vi "LaserToBuffer.vi"() -> ()   [LabVIEW 2016]
uses:
  <instrlib>/Keyence LK-G3000/Public/clusters/LKIF_FLOATVALUE.ctl
  <instrlib>/Keyence LK-G3000/Public/enums/LKIF_FLOATRESULT.ctl
  <instrlib>/Keyence LK-G3000/Keyence LK-G3000.lvlib
panel:
  in  "timing":u32=500
  out "Measurements":dbl[][](array[numeric])
  out "CalcData2":T1 {"LKIF_FLOATRESULT" items=["VALID", "RANGEOVER_P", "RANGEOVER_N", "WAITING"]}
  out "CalcData1":T1 {"LKIF_FLOATRESULT" items=["VALID", "RANGEOVER_P", "RANGEOVER_N", "WAITING"]}
  in  "Stop VI":bool
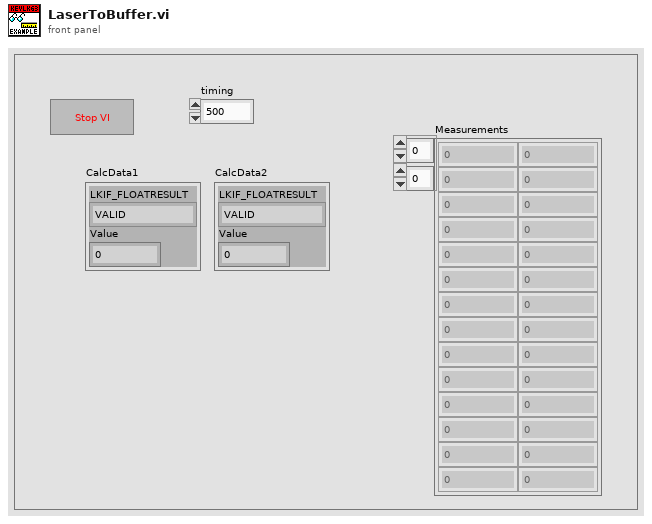
[diagram p1: front panel]
types:
  T1 = typedef "Keyence LK-G3000.lvlib/LKIF_FLOATVALUE.ctl" = cluster{"LKIF_FLOATRESULT":T2, "Value":sgl}
  T2 = typedef "Keyence LK-G3000.lvlib/LKIF_FLOATRESULT.ctl" = i32
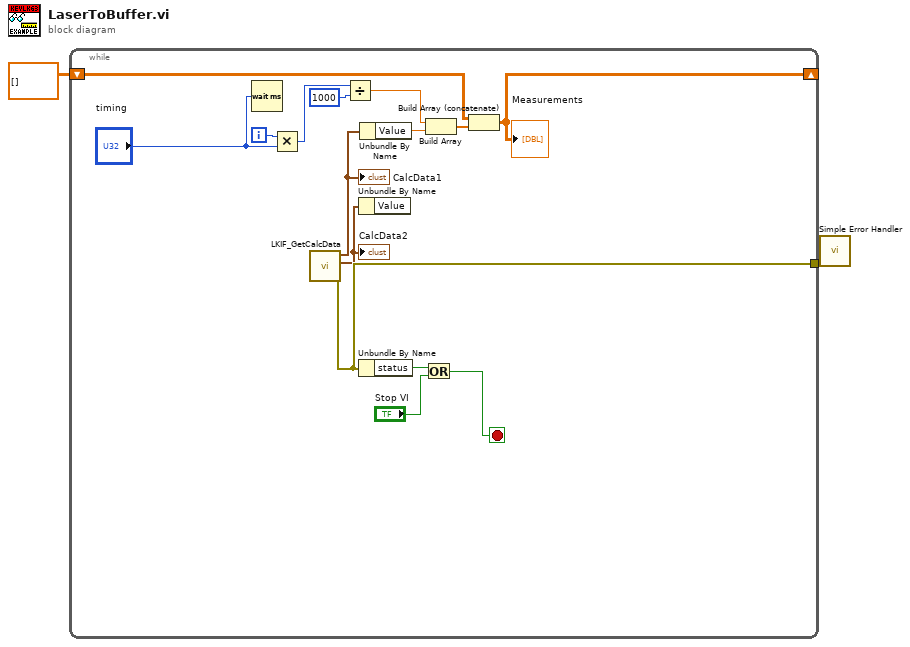
[diagram p0: block diagram]
diagram:
  n1 = while {
    tunnel: [w17] -> w2
    shift-right: [w11] -> _
    shift-left: dbl[][] [] -> [w12]
    i -> [w10]
    stop <- w3 stop-if-true
    n2 = Wait (ms)(milliseconds to wait="timing") -> ()  [unwired: 1 out]
    n3 = Multiply(x=w10, y="timing") -> (x*y=w6:u32)
    n4 = call <instrlib>:"LKIF_GetCalcData.vi"() -> ("error out"=w17:errorcluster, "CalcData2"=w13:T1, "CalcData1"=w14:T1)  [unwired: 9 in]
    "CalcData1" <- w14
    "CalcData2" <- w13
    n5 = Divide(x=w6, y=1000) -> (x/y=w4:dbl)
    n6 = Unbundle By Name(w13) -> ()  [unwired: 1 out]
    n7 = Unbundle By Name(w17) -> ("status"=w16:bool)
    n8 = Unbundle By Name(w14) -> ("Value"=w8:sgl)
    n9 = Or(x=w16, y="Stop VI") -> (x .or. y?=w3:bool)
    n10 = Build Array(w4, w8) -> (w9:dbl[])
    n11 = Build Array (concatenate)(w12, w9) -> (w11:dbl[][])
    "Measurements" <- w11
  }
  n12 = call <vilib>:"Simple Error Handler.vi"("error in (no error)"=w2) -> ()  [unwired: 4 in, 5 out]
